vi "CAN Filter Messages.vi"(7 "Mode":u8, 8 "error in (no error)":errorcluster, 9 "ToID":u32, 10 "FromID":u32, 11 "Channel":u16) -> (0 "error out":errorcluster, 2 "Channel out":u16, 3 "function return":u32)   [LabVIEW 2023, in "PCAN2023.lvlib"]
doc: "The message filter will be expanded with every call to this function. If it is desired to reset the filter, please use the 'SetValue' function\n\n\nTPCANStatus __stdcall CAN_FilterMessages(\n TPCANHandle Channel, \n DWORD FromID, \n DWORD ToID, \n TPCANMode Mode);"
uses:
  PCAN2023.lvlib
  PCANBasic.dll
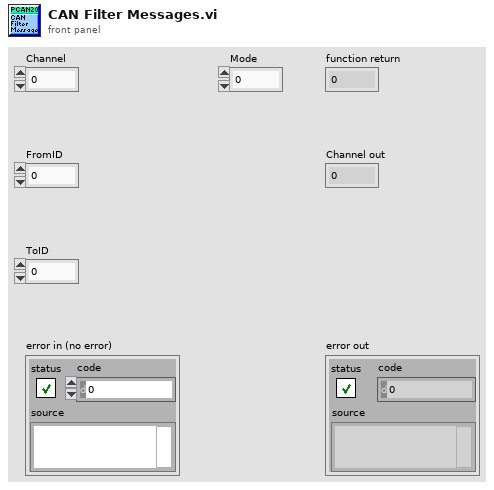
[diagram p1: front panel]
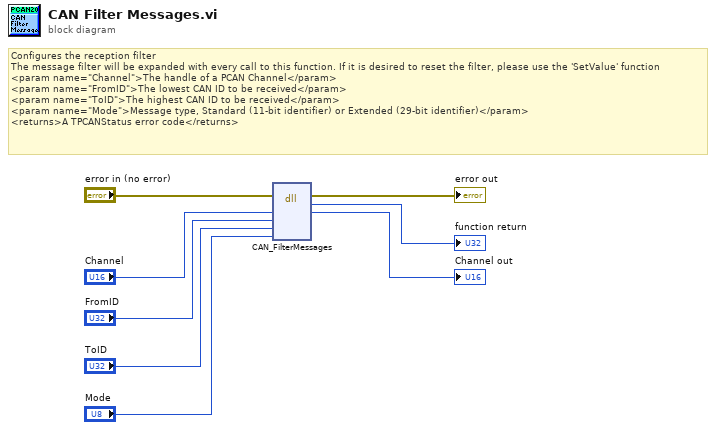
[diagram p0: block diagram]
diagram:
  # "Configures the reception filter\nThe message filter will be expanded with every call to this function. If it is desired to reset the filter, please use the 'SetValue' function\n<param name=\"Channel\">The handle of a PCAN Channel</param>\n<param name=\"FromID\">The lowest CAN ID to be received</param>\n<param name=\"ToID\">The highest CAN ID to be received</param>\n<param name=\"Mode\">Message type, Standard (11-bit identifier) or Extended (29-bit identifier)</param>\n<returns>A TPCANStatus error code</returns>"
  n1 = dll-call lib="D:/PEAK/PCAN2023/PCAN2023/PCANBasic.*" fn="CAN_FilterMessages"(error in="error in (no error)", "Channel"="Channel", "FromID"="FromID", "ToID"="ToID", "Mode"="Mode") -> (error out=→"error out":errorcluster, →"function return":u32, "Channel"=→"Channel out":u16)  [unwired: 5 in, 1 out]
